vi "MDAQ_PrepCVArray.vi"(9 "input cluster":T3 {"CV"."Temperature Array" scale=0.0..100.0}, 10 "Concurrent CV Arrays":T1, 11 "Status_Cluster":T2 {"GATESTOP" format="%04x"; "GATESTRT" format="%04x"; "AMPLITUDE" format="%04x"; "M_CYCLES" format="%04x"; "N_CYCLES" format="%04x"; "STEP" format="%04x"; "BASE" format="%04x"; "CHAN" format="%04x"}) -> (1 "Output cluster":T3 {"CV"."Temperature Array" scale=0.0..100.0}, 2 "Concurrent CV Arrays Out":T1, 3 "Status_Cluster Out":T2 {"GATESTOP" format="%04x"; "GATESTRT" format="%04x"; "AMPLITUDE" format="%04x"; "M_CYCLES" format="%04x"; "N_CYCLES" format="%04x"; "STEP" format="%04x"; "BASE" format="%04x"; "CHAN" format="%04x"})   [LabVIEW 2021]
uses:
  GUI_Def.ctl
  Mode_Enum.ctl
  Status_Cluster.ctl
  Array_Cluster.ctl
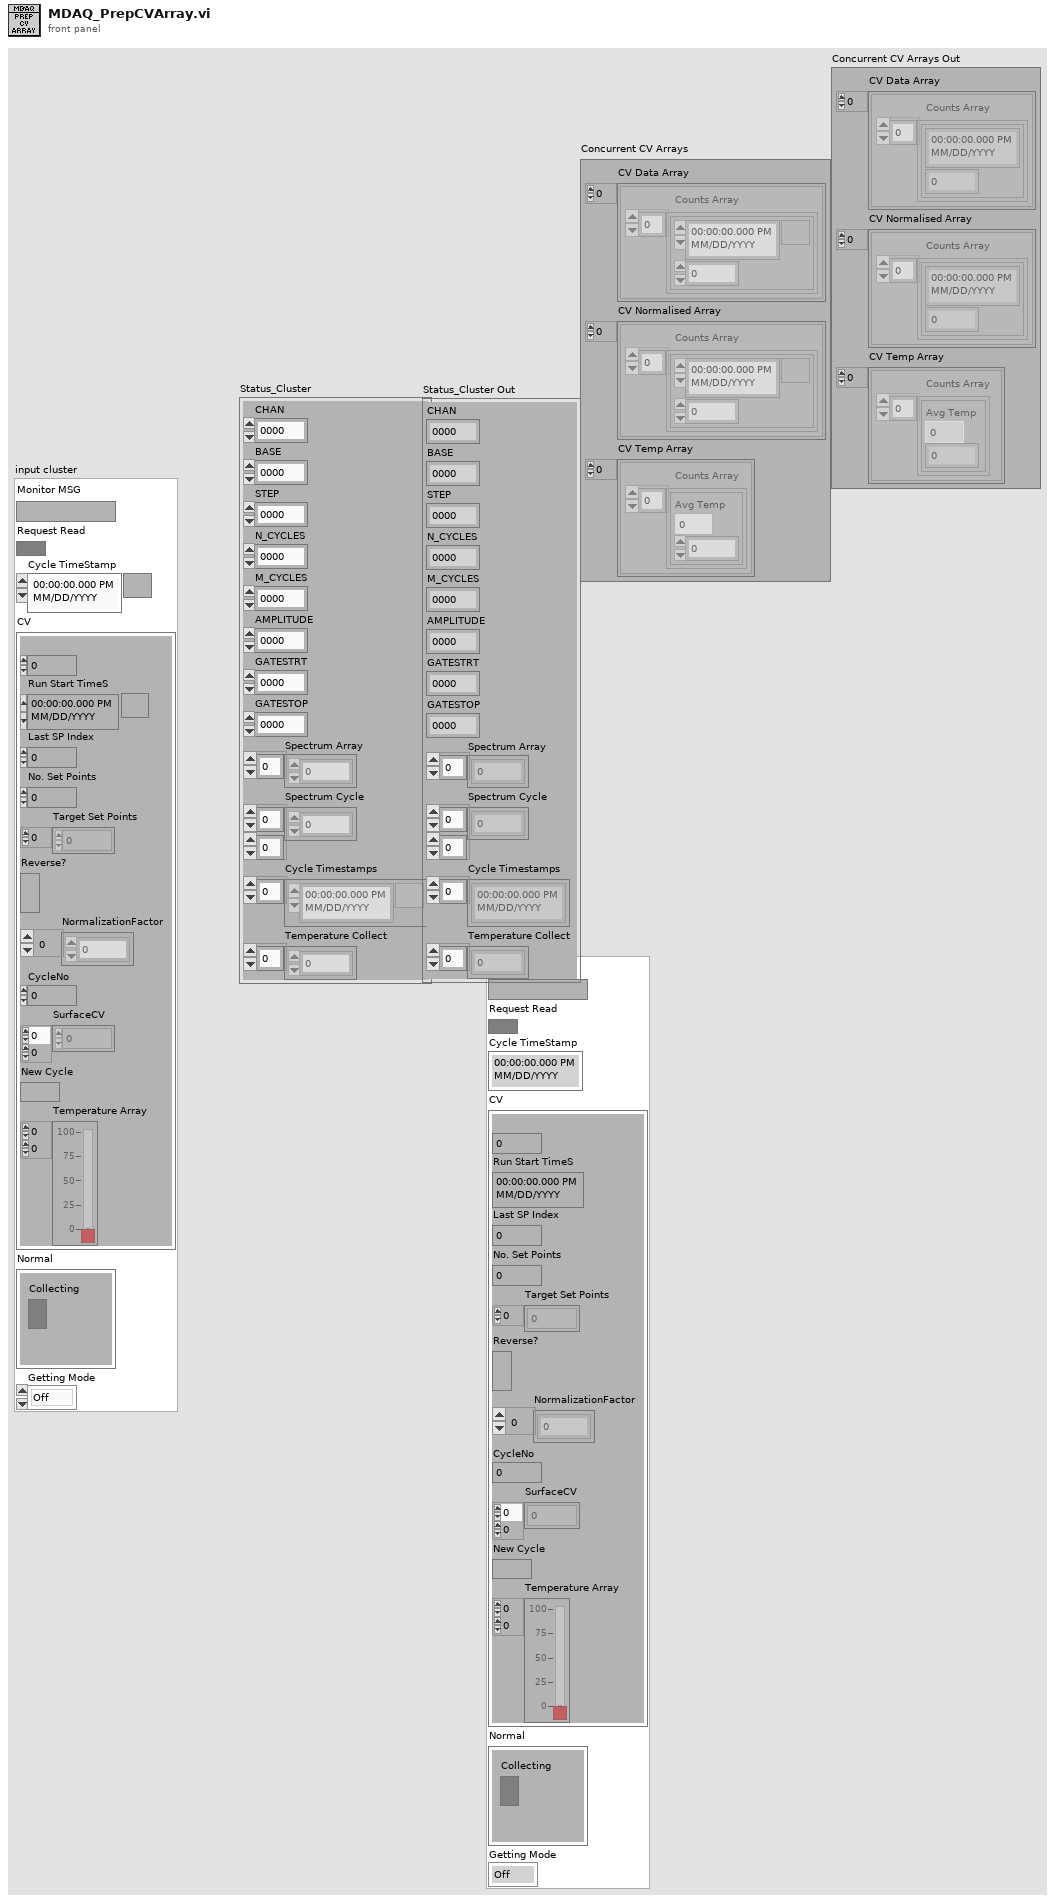
[diagram p1: front panel]
types:
  T1 = typedef "Array_Cluster.ctl" = cluster{"CV Data Array":cluster{"Counts Array":cluster{timestamp, i32}[]}[], "CV Normalised Array":cluster{"Counts Array":cluster{timestamp, dbl}[]}[], "CV Temp Array":cluster{"Counts Array":cluster{"Avg Temp":dbl, dbl}[]}[]}
  T2 = typedef "Status_Cluster.ctl" = cluster{"CHAN":u32, "BASE":u32, "STEP":u32, "N_CYCLES":u32, "M_CYCLES":u32, "AMPLITUDE":u32, "GATESTRT":u32, "GATESTOP":u32, "Spectrum Array":u32[], "Spectrum Cycle":u32[][], "Cycle Timestamps":timestamp[], "Temperature Collect":dbl[]}
  T3 = typedef "GUI_Def.ctl" = cluster{"Monitor MSG":string, "Request Read":bool, "Cycle TimeStamp":timestamp, "CV":cluster{"Set Point Index":u32, "Run Start TimeS":timestamp, "Last SP Index":u32, "No. Set Points":u32, "Target Set Points":i32[], "Reverse?":bool, "NormalizationFactor":i32[], "CycleNo":i32, "SurfaceCV":dbl[][], "New Cycle":bool, "Temperature Array":dbl[][]}, "Normal":cluster{"Collecting":bool}, "Getting Mode":T4}
  T4 = typedef "Mode_Enum.ctl" = enum16{"Off", "Normal", "CV+Temp", "CV"}
  T5 = cluster{"Counts Array":cluster{"Avg Temp":dbl, dbl}[]}[]
  T6 = cluster{"Counts Array":cluster{"Avg Temp":dbl, dbl}[]}
  T7 = cluster{"Counts Array":cluster{timestamp, dbl}[]}[]
  T8 = cluster{"BackgroundArray":cluster{timestamp, i32}[]}[]
  T9 = cluster{"Counts Array":cluster{timestamp, dbl}[]}
  T10 = cluster{"BackgroundArray":cluster{timestamp, i32}[]}
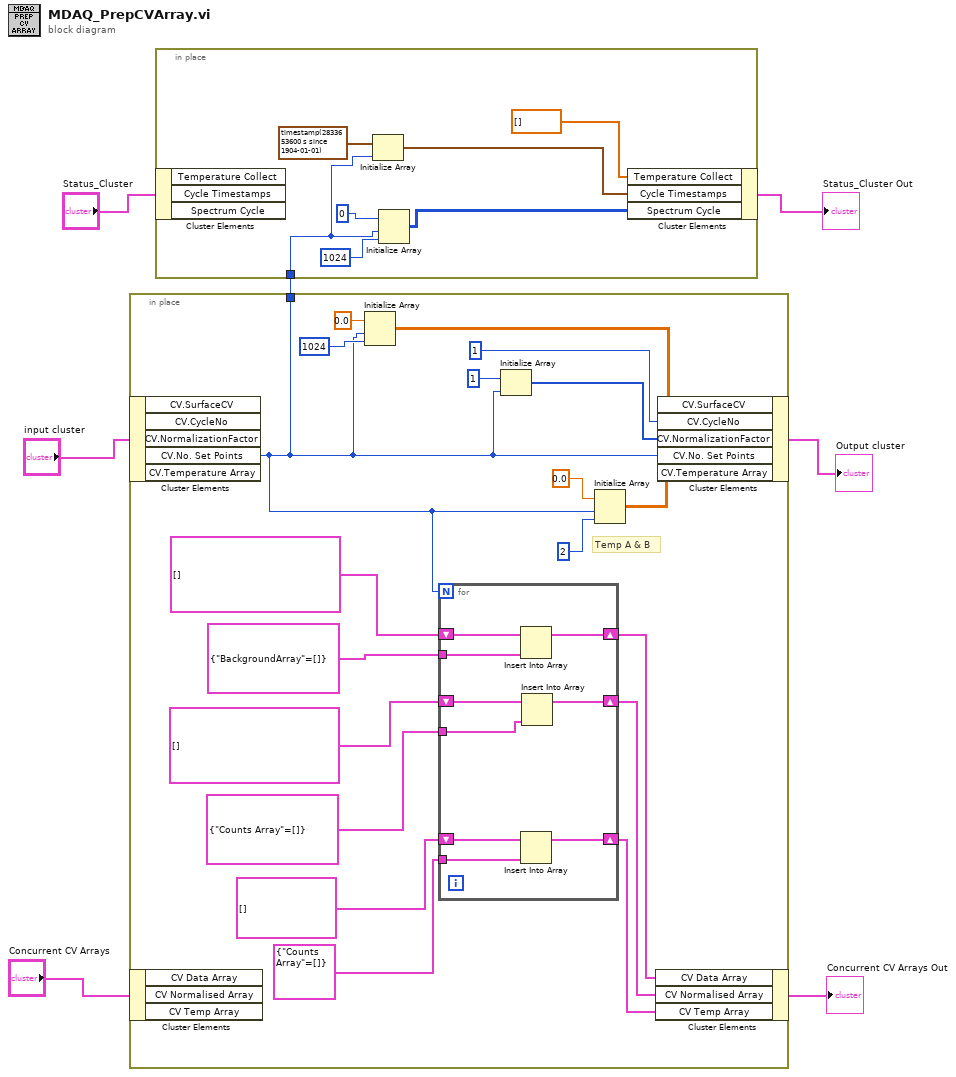
[diagram p0: block diagram]
diagram:
  n1 = in-place {
    in-place-border: [w15] -> w4
    # "Temp A & B"
    n2 = in-place-cluster #1("input cluster") -> ("CV.No. Set Points"=w15:u32)  [unwired: 4 out]
    n3 = in-place-cluster #2("Concurrent CV Arrays") -> ()  [unwired: 3 out]
    n4 = Initialize Array(0.0 ("element"), w15, 1024 ("dimension size")) -> (w18:dbl[][])
    n5 = for {
      N: w15 -> [_]
      shift-right: [w34] -> w12
      shift-left: T8 [] -> [w35]
      tunnel: T10 {"BackgroundArray"=[]} ("new element/subarray") -> [w33]
      shift-right: [w31] -> w11
      shift-left: T7 [] -> [w32]
      tunnel: T9 {"Counts Array"=[]} ("new element/subarray") -> [w30]
      shift-right: [w28] -> w10
      shift-left: T5 [] ("CV Temp Array") -> [w29]
      tunnel: T6 {"Counts Array"=[]} ("Spectrum Array") -> [w27]
      n6 = Insert Into Array(array=w35, new element=w33) -> (w34:T8)  [unwired: 1 in]
      n7 = Insert Into Array(array=w29, new element=w27) -> (w28:T5)  [unwired: 1 in]
      n8 = Insert Into Array(array=w32, new element=w30) -> (w31:T7)  [unwired: 1 in]
    }
    n9 = Initialize Array(1, w15) -> (w22:i32[])
    n10 = Initialize Array(0.0 ("element"), w15, 2 ("dimension size")) -> (w16:dbl[][])
    n11 = in-place-cluster #2("CV Data Array"=w12, "CV Normalised Array"=w11, "CV Temp Array"=w10) -> (→"Concurrent CV Arrays Out":T1)
    n12 = in-place-cluster #1("CV.SurfaceCV"=w18, "CV.CycleNo"=1, "CV.NormalizationFactor"=w22, "CV.No. Set Points"=w15, "CV.Temperature Array"=w16) -> (→"Output cluster":T3)
  }
  n13 = in-place {
    in-place-border: w4 -> [w37]
    n14 = in-place-cluster #3("Status_Cluster") -> ()  [unwired: 3 out]
    n15 = Initialize Array(timestamp(2833653600 s since 1904-01-01), w37) -> (w38:timestamp[])
    n16 = Initialize Array(u32 0, w37, 1024 ("dimension size")) -> (w40:u32[][])
    n17 = in-place-cluster #3("Temperature Collect"=dbl[] [], "Cycle Timestamps"=w38, "Spectrum Cycle"=w40) -> (→"Status_Cluster Out":T2)
  }
